vi "initialiseDevice.vi"(8 "error in (no error)":errorcluster, 10 "deviceName":string, 11 "AtomChipHWC in":refnum<class "AtomChipHWC.lvclass">) -> (0 "error out":errorcluster, 3 "AtomChipHWC out":refnum<class "AtomChipHWC.lvclass">)   [LabVIEW 2009, in "Hardware.lvlib" / "HWControllers.lvlib" / "AtomChipHWC.lvclass"]
doc: "Initialise a hardware device. \nI.e. set its initial channel states etc."
uses:
  AtomChipHWC.lvclass
  AtomChipHWC.lvclass/AtomChipHWC.ctl
  Channels/VoltOutput/AnalogOutput.lvclass
  Channels/Digital/DigitalOutput.lvclass
  Channels/DDSOutput/Generic/DDSOutput.lvclass
  Network Controllers/NetworkCamera/NetworkCamera.lvclass
  HWController.lvclass
  Tools/DatabaseHelpers/DbConnection/DeviceDataBase/deviceDataBase.lvclass
  Network Controllers/CameraNetworkController/CameraNetworkController.lvclass
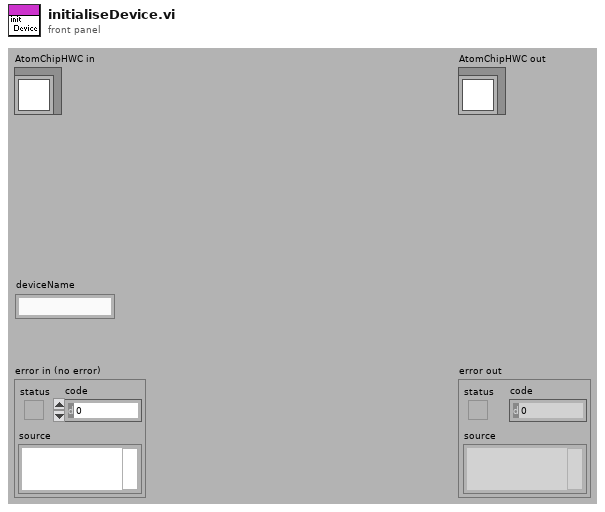
[diagram p1: front panel]
types:
  T1 = cluster{"Frequency(MHz)":dbl, "Amplitude":dbl, "Phase":dbl, "OutputForm":enum16{"Sine", "Square", "Triangle", "Arbitrary"}}[]
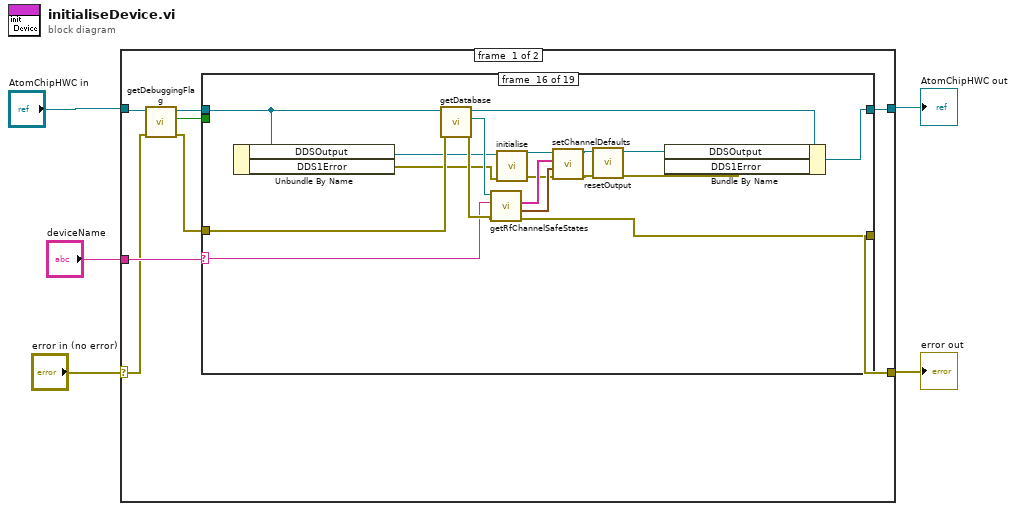
[diagram p0: block diagram]
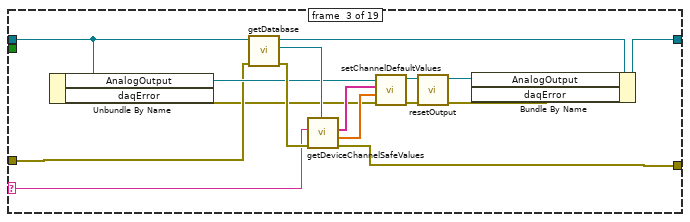
[diagram p4: hidden frame]
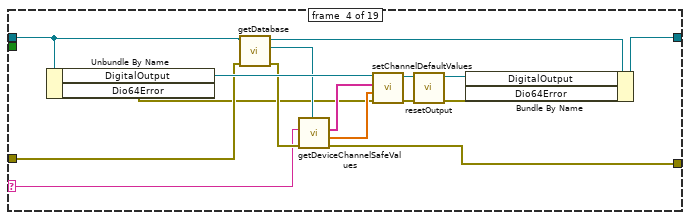
[diagram p5: hidden frame]
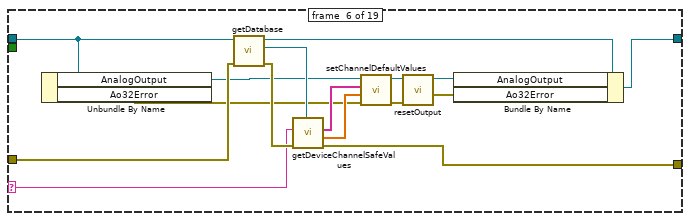
[diagram p7: hidden frame]
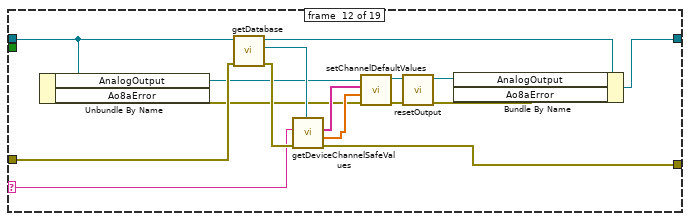
[diagram p13: hidden frame]
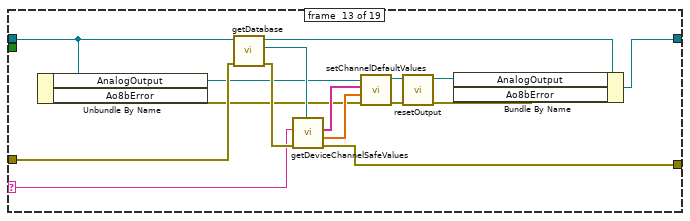
[diagram p14: hidden frame]
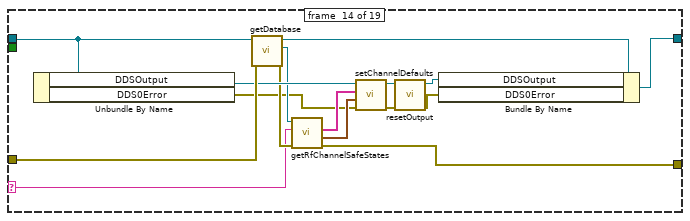
[diagram p15: hidden frame]
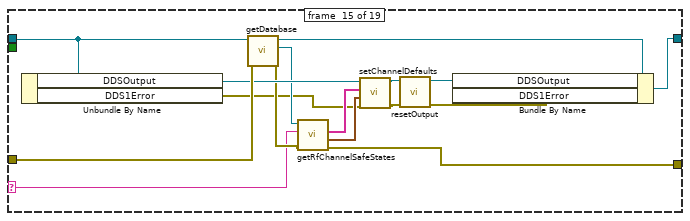
[diagram p16: hidden frame]
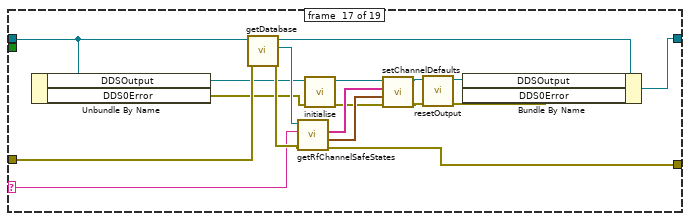
[diagram p17: hidden frame]
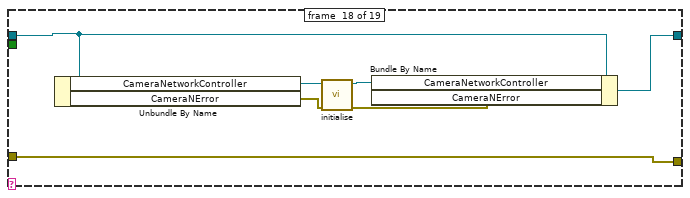
[diagram p18: hidden frame]
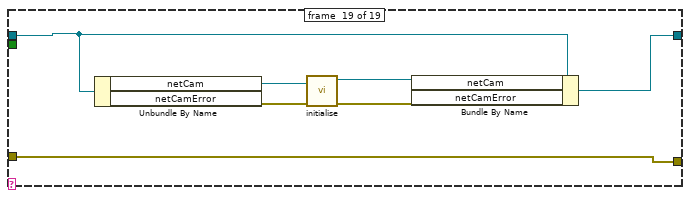
[diagram p19: hidden frame]
diagram:
  n1 = case shown="No Error" "error in (no error)" {
    selector: "error in (no error)" -> [w8 w193]
    tunnel: [w11 w193] -> w4
    tunnel: [w13 w192] -> w2
    tunnel: "AtomChipHWC in" -> [w10 w192]
    tunnel: "deviceName" -> [w12 _]
    frame #0 {
      n2 = call "getDebuggingFlag.vi"("error in (no error)"=w8, "HWController.lvclass in"=w10) -> ("error out"=w7:errorcluster, "debuggingFlag"=w6:bool, "HWController.lvclass out"=w9:refnum<class "AtomChipHWC.lvclass">)  [unwired: 7 in]
      n3 = case shown="\"k3390\"" w12 {
        selector: w12 -> [_ _ w21 w40 _ w65 _ _ _ _ _ w91 w107 w118 w135 w154 w172 _ _]
        tunnel: w9 -> [w15 w17 w24 w44 w50 w59 w69 w71 w73 w75 w77 w86 w101 w124 w140 w158 w176 w183 w191]
        tunnel: [w15 w17 w22 w45 w50 w55 w69 w71 w73 w75 w77 w82 w97 w122 w138 w156 w174 w181 w190] -> w13
        tunnel: w7 -> [w14 w16 w23 w37 w51 w64 w68 w70 w72 w74 w76 w90 w106 w125 w141 w159 w177 w178 w189]
        tunnel: [w14 w16 w18 w34 w51 w52 w68 w70 w72 w74 w76 w79 w96 w112 w128 w147 w165 w178 w189] -> w11
        tunnel: w6 -> [_ _ _ _ _ _ _ _ _ _ _ _ _ _ _ _ _ _ _]
        frame #0 {
        }
        frame #1 {
        }
        frame #2 {
          n4 = Unbundle By Name(w24) -> ("AnalogOutput"=w27:refnum<class "AnalogOutput.lvclass">, "daqError"=w20:errorcluster)
          n5 = call "getDatabase.vi"("error in (no error)"=w23, "HWController in"=w24) -> ("error out"=w32:errorcluster, "deviceDataBase"=w33:refnum<class "deviceDataBase.lvclass">, "HWController out"=w25:refnum<class "AtomChipHWC.lvclass">)  [unwired: 7 in]
          n6 = call "getDeviceChannelSafeValues.vi"("error in (no error)"=w32, "device_name"=w21, "deviceDataBase in"=w33) -> ("error out"=w18:errorcluster, "SafeVaues"=w31:dbl[], "ChannelAddresses"=w30:string[])  [unwired: 5 in, 1 out]
          n7 = call "setChannelDefaultValues.vi"("error in (no error)"=w20, "calibratedValues"=w31, "channel_addresses"=w30, "AnalogOutput in"=w27) -> ("error out"=w28:errorcluster, "AnalogOutput out"=w29:refnum<class "AnalogOutput.lvclass">)  [unwired: 6 in]
          n8 = call-dynamic "resetOutput.vi"("error in (no error)"=w28, "AnalogOutput in"=w29) -> ("error out"=w19:errorcluster, "AnalogOutput out"=w26:refnum<class "AnalogOutput.lvclass">)  [unwired: 8 in]
          n9 = Bundle By Name(cluster=w25, "AnalogOutput"=w26, "daqError"=w19) -> (w22:refnum<class "AtomChipHWC.lvclass">)
        }
        frame #3 {
          n10 = Unbundle By Name(w44) -> ("DigitalOutput"=w49:refnum<class "DigitalOutput.lvclass">, "Dio64Error"=w36:errorcluster)
          n11 = call "getDatabase.vi"("error in (no error)"=w37, "HWController in"=w44) -> ("error out"=w41:errorcluster, "deviceDataBase"=w42:refnum<class "deviceDataBase.lvclass">, "HWController out"=w43:refnum<class "AtomChipHWC.lvclass">)  [unwired: 7 in]
          n12 = call "getDeviceChannelSafeValues.vi"("error in (no error)"=w41, "device_name"=w40, "deviceDataBase in"=w42) -> ("error out"=w34:errorcluster, "SafeVaues"=w38:dbl[], "ChannelAddresses"=w39:string[])  [unwired: 5 in, 1 out]
          n13 = call-dynamic "setChannelDefaultValues.vi"("error in (no error)"=w36, "calibratedValues"=w38, "channel_addresses"=w39, "DigitalOutput in"=w49) -> ("error out"=w47:errorcluster, "DigitalOutput out"=w48:refnum<class "DigitalOutput.lvclass">)  [unwired: 6 in]
          n14 = call-dynamic "resetOutput.vi"("error in (no error)"=w47, "DigitalOutput in"=w48) -> ("error out"=w35:errorcluster, "DigitalOutput out"=w46:refnum<class "DigitalOutput.lvclass">)  [unwired: 8 in]
          n15 = Bundle By Name(cluster=w43, "DigitalOutput"=w46, "Dio64Error"=w35) -> (w45:refnum<class "AtomChipHWC.lvclass">)
        }
        frame #4 {
        }
        frame #5 {
          n16 = Unbundle By Name(w59) -> ("AnalogOutput"=w58:refnum<class "AnalogOutput.lvclass">, "Ao32Error"=w54:errorcluster)
          n17 = call "getDatabase.vi"("error in (no error)"=w64, "HWController in"=w59) -> ("error out"=w66:errorcluster, "deviceDataBase"=w67:refnum<class "deviceDataBase.lvclass">, "HWController out"=w56:refnum<class "AtomChipHWC.lvclass">)  [unwired: 7 in]
          n18 = call "getDeviceChannelSafeValues.vi"("error in (no error)"=w66, "device_name"=w65, "deviceDataBase in"=w67) -> ("error out"=w52:errorcluster, "SafeVaues"=w63:dbl[], "ChannelAddresses"=w62:string[])  [unwired: 5 in, 1 out]
          n19 = call "setChannelDefaultValues.vi"("error in (no error)"=w54, "calibratedValues"=w63, "channel_addresses"=w62, "AnalogOutput in"=w58) -> ("error out"=w60:errorcluster, "AnalogOutput out"=w61:refnum<class "AnalogOutput.lvclass">)  [unwired: 6 in]
          n20 = call-dynamic "resetOutput.vi"("error in (no error)"=w60, "AnalogOutput in"=w61) -> ("error out"=w53:errorcluster, "AnalogOutput out"=w57:refnum<class "AnalogOutput.lvclass">)  [unwired: 8 in]
          n21 = Bundle By Name(cluster=w56, "AnalogOutput"=w57, "Ao32Error"=w53) -> (w55:refnum<class "AtomChipHWC.lvclass">)
        }
        frame #6 {
        }
        frame #7 {
        }
        frame #8 {
        }
        frame #9 {
        }
        frame #10 {
        }
        frame #11 {
          n22 = Unbundle By Name(w86) -> ("AnalogOutput"=w85:refnum<class "AnalogOutput.lvclass">, "Ao8aError"=w80:errorcluster)
          n23 = call "getDatabase.vi"("error in (no error)"=w90, "HWController in"=w86) -> ("error out"=w92:errorcluster, "deviceDataBase"=w93:refnum<class "deviceDataBase.lvclass">, "HWController out"=w83:refnum<class "AtomChipHWC.lvclass">)  [unwired: 7 in]
          n24 = call "getDeviceChannelSafeValues.vi"("error in (no error)"=w92, "device_name"=w91, "deviceDataBase in"=w93) -> ("error out"=w79:errorcluster, "SafeVaues"=w81:dbl[], "ChannelAddresses"=w89:string[])  [unwired: 5 in, 1 out]
          n25 = call "setChannelDefaultValues.vi"("error in (no error)"=w80, "calibratedValues"=w81, "channel_addresses"=w89, "AnalogOutput in"=w85) -> ("error out"=w87:errorcluster, "AnalogOutput out"=w88:refnum<class "AnalogOutput.lvclass">)  [unwired: 6 in]
          n26 = call-dynamic "resetOutput.vi"("error in (no error)"=w87, "AnalogOutput in"=w88) -> ("error out"=w78:errorcluster, "AnalogOutput out"=w84:refnum<class "AnalogOutput.lvclass">)  [unwired: 8 in]
          n27 = Bundle By Name(cluster=w83, "AnalogOutput"=w84, "Ao8aError"=w78) -> (w82:refnum<class "AtomChipHWC.lvclass">)
        }
        frame #12 {
          n28 = Unbundle By Name(w101) -> ("AnalogOutput"=w100:refnum<class "AnalogOutput.lvclass">, "Ao8bError"=w94:errorcluster)
          n29 = call "getDatabase.vi"("error in (no error)"=w106, "HWController in"=w101) -> ("error out"=w108:errorcluster, "deviceDataBase"=w109:refnum<class "deviceDataBase.lvclass">, "HWController out"=w98:refnum<class "AtomChipHWC.lvclass">)  [unwired: 7 in]
          n30 = call "getDeviceChannelSafeValues.vi"("error in (no error)"=w108, "device_name"=w107, "deviceDataBase in"=w109) -> ("error out"=w96:errorcluster, "SafeVaues"=w105:dbl[], "ChannelAddresses"=w104:string[])  [unwired: 5 in, 1 out]
          n31 = call "setChannelDefaultValues.vi"("error in (no error)"=w94, "calibratedValues"=w105, "channel_addresses"=w104, "AnalogOutput in"=w100) -> ("error out"=w102:errorcluster, "AnalogOutput out"=w103:refnum<class "AnalogOutput.lvclass">)  [unwired: 6 in]
          n32 = call-dynamic "resetOutput.vi"("error in (no error)"=w102, "AnalogOutput in"=w103) -> ("error out"=w95:errorcluster, "AnalogOutput out"=w99:refnum<class "AnalogOutput.lvclass">)  [unwired: 8 in]
          n33 = Bundle By Name(cluster=w98, "AnalogOutput"=w99, "Ao8bError"=w95) -> (w97:refnum<class "AtomChipHWC.lvclass">)
        }
        frame #13 {
          n34 = Unbundle By Name(w124) -> ("DDSOutput"=w121:refnum<class "DDSOutput.lvclass">, "DDS0Error"=w111:errorcluster)
          n35 = call "getDatabase.vi"("error in (no error)"=w125, "HWController in"=w124) -> ("error out"=w120:errorcluster, "deviceDataBase"=w119:refnum<class "deviceDataBase.lvclass">, "HWController out"=w123:refnum<class "AtomChipHWC.lvclass">)  [unwired: 7 in]
          n36 = call "getRfChannelSafeStates.vi"("error in (no error)"=w120, "deviceName"=w118, "deviceDataBase in"=w119) -> ("error out"=w112:errorcluster, "safestates"=w113:T1, "ChannelAddresses"=w114:string[])  [unwired: 5 in, 1 out]
          n37 = call-dynamic "setChannelDefaults.vi"("error in (no error)"=w111, "Data"=w113, "physicalChannels"=w114, "DDSOutput in"=w121) -> ("error out"=w115:errorcluster, "DDSOutput out"=w117:refnum<class "DDSOutput.lvclass">)  [unwired: 6 in]
          n38 = call-dynamic "resetOutput.vi"("error in (no error)"=w115, "DDSOutput in"=w117) -> ("error out"=w110:errorcluster, "DDSOutput out"=w116:refnum<class "DDSOutput.lvclass">)  [unwired: 8 in]
          n39 = Bundle By Name(cluster=w123, "DDSOutput"=w116, "DDS0Error"=w110) -> (w122:refnum<class "AtomChipHWC.lvclass">)
        }
        frame #14 {
          n40 = Unbundle By Name(w140) -> ("DDSOutput"=w137:refnum<class "DDSOutput.lvclass">, "DDS1Error"=w127:errorcluster)
          n41 = call "getDatabase.vi"("error in (no error)"=w141, "HWController in"=w140) -> ("error out"=w136:errorcluster, "deviceDataBase"=w134:refnum<class "deviceDataBase.lvclass">, "HWController out"=w139:refnum<class "AtomChipHWC.lvclass">)  [unwired: 7 in]
          n42 = call "getRfChannelSafeStates.vi"("error in (no error)"=w136, "deviceName"=w135, "deviceDataBase in"=w134) -> ("error out"=w128:errorcluster, "safestates"=w132:T1, "ChannelAddresses"=w133:string[])  [unwired: 5 in, 1 out]
          n43 = call-dynamic "setChannelDefaults.vi"("error in (no error)"=w127, "Data"=w132, "physicalChannels"=w133, "DDSOutput in"=w137) -> ("error out"=w129:errorcluster, "DDSOutput out"=w131:refnum<class "DDSOutput.lvclass">)  [unwired: 6 in]
          n44 = call-dynamic "resetOutput.vi"("error in (no error)"=w129, "DDSOutput in"=w131) -> ("error out"=w126:errorcluster, "DDSOutput out"=w130:refnum<class "DDSOutput.lvclass">)  [unwired: 8 in]
          n45 = Bundle By Name(cluster=w139, "DDSOutput"=w130, "DDS1Error"=w126) -> (w138:refnum<class "AtomChipHWC.lvclass">)
        }
        frame #15 {
          n46 = Unbundle By Name(w158) -> ("DDSOutput"=w144:refnum<class "DDSOutput.lvclass">, "DDS1Error"=w142:errorcluster)
          n47 = call "getDatabase.vi"("error in (no error)"=w159, "HWController in"=w158) -> ("error out"=w155:errorcluster, "deviceDataBase"=w153:refnum<class "deviceDataBase.lvclass">, "HWController out"=w157:refnum<class "AtomChipHWC.lvclass">)  [unwired: 7 in]
          n48 = call "getRfChannelSafeStates.vi"("error in (no error)"=w155, "deviceName"=w154, "deviceDataBase in"=w153) -> ("error out"=w147:errorcluster, "safestates"=w151:T1, "ChannelAddresses"=w152:string[])  [unwired: 5 in, 1 out]
          n49 = call-dynamic "initialise.vi"("error in (no error)"=w142, "DDSOutput in"=w144) -> ("error out"=w143:errorcluster, "DDSOutput out"=w145:refnum<class "DDSOutput.lvclass">)  [unwired: 8 in]
          n50 = call-dynamic "setChannelDefaults.vi"("error in (no error)"=w143, "Data"=w151, "physicalChannels"=w152, "DDSOutput in"=w145) -> ("error out"=w148:errorcluster, "DDSOutput out"=w150:refnum<class "DDSOutput.lvclass">)  [unwired: 6 in]
          n51 = call-dynamic "resetOutput.vi"("error in (no error)"=w148, "DDSOutput in"=w150) -> ("error out"=w146:errorcluster, "DDSOutput out"=w149:refnum<class "DDSOutput.lvclass">)  [unwired: 8 in]
          n52 = Bundle By Name(cluster=w157, "DDSOutput"=w149, "DDS1Error"=w146) -> (w156:refnum<class "AtomChipHWC.lvclass">)
        }
        frame #16 {
          n53 = Unbundle By Name(w176) -> ("DDSOutput"=w162:refnum<class "DDSOutput.lvclass">, "DDS0Error"=w160:errorcluster)
          n54 = call "getDatabase.vi"("error in (no error)"=w177, "HWController in"=w176) -> ("error out"=w173:errorcluster, "deviceDataBase"=w171:refnum<class "deviceDataBase.lvclass">, "HWController out"=w175:refnum<class "AtomChipHWC.lvclass">)  [unwired: 7 in]
          n55 = call "getRfChannelSafeStates.vi"("error in (no error)"=w173, "deviceName"=w172, "deviceDataBase in"=w171) -> ("error out"=w165:errorcluster, "safestates"=w169:T1, "ChannelAddresses"=w170:string[])  [unwired: 5 in, 1 out]
          n56 = call-dynamic "initialise.vi"("error in (no error)"=w160, "DDSOutput in"=w162) -> ("error out"=w161:errorcluster, "DDSOutput out"=w163:refnum<class "DDSOutput.lvclass">)  [unwired: 8 in]
          n57 = call-dynamic "setChannelDefaults.vi"("error in (no error)"=w161, "Data"=w169, "physicalChannels"=w170, "DDSOutput in"=w163) -> ("error out"=w166:errorcluster, "DDSOutput out"=w168:refnum<class "DDSOutput.lvclass">)  [unwired: 6 in]
          n58 = call-dynamic "resetOutput.vi"("error in (no error)"=w166, "DDSOutput in"=w168) -> ("error out"=w164:errorcluster, "DDSOutput out"=w167:refnum<class "DDSOutput.lvclass">)  [unwired: 8 in]
          n59 = Bundle By Name(cluster=w175, "DDSOutput"=w167, "DDS0Error"=w164) -> (w174:refnum<class "AtomChipHWC.lvclass">)
        }
        frame #17 {
          n60 = Unbundle By Name(w183) -> ("CameraNetworkController"=w184:refnum<class "CameraNetworkController.lvclass">, "CameraNError"=w180:errorcluster)
          n61 = call "initialise.vi"("error in (no error)"=w180, "CameraNetworkController in"=w184) -> ("error out"=w179:errorcluster, "CameraNetworkController out"=w182:refnum<class "CameraNetworkController.lvclass">)  [unwired: 8 in]
          n62 = Bundle By Name(cluster=w183, "CameraNetworkController"=w182, "CameraNError"=w179) -> (w181:refnum<class "AtomChipHWC.lvclass">)
        }
        frame #18 {
          n63 = Unbundle By Name(w191) -> ("netCam"=w188:refnum<class "NetworkCamera.lvclass">, "netCamError"=w186:errorcluster)
          n64 = call-dynamic "initialise.vi"("error in (no error)"=w186, "NetworkCamera in"=w188) -> ("error out"=w185:errorcluster, "NetworkCamera out"=w187:refnum<class "NetworkCamera.lvclass">)  [unwired: 8 in]
          n65 = Bundle By Name(cluster=w191, "netCam"=w187, "netCamError"=w185) -> (w190:refnum<class "AtomChipHWC.lvclass">)
        }
      }
    }
    frame #1 {
    }
  }
  "error out" <- w4
  "AtomChipHWC out" <- w2
